vi "Log Messages.vi"(8 "error in (no error)":errorcluster, 10 "Actor to Log":refnum<class "Message Enqueuer.lvclass">, 11 "Monitor in":refnum<class "Classic Monitor.lvclass">) -> (0 "error out":errorcluster, 3 "Monitor out":refnum<class "Classic Monitor.lvclass">)   [LabVIEW 2023, in "Monitored Actor.lvlib" / "Classic Monitor.lvclass"]
doc: "Starts message logging on the specified actor\n\nCopyright: MGI 2016\nAuthor: Derek Trepanier"
uses:
  Classic Monitor.lvclass
  C:/Users/Public/Documents/Development/Framework/Monitored Actor/Actor Monitor/Actor Monitor/Actor Monitor.lvclass
  C:/Users/Public/Documents/Development/builds/Framework/Actor Framework.lvlibp/1abvi3w/vi.lib/ActorFramework/Actor/Actor.lvclass
  builds/Framework/Actor Framework.lvlibp/1abvi3w/vi.lib/ActorFramework/Message Enqueuer/Message Enqueuer.lvclass
  Actor Monitor/Actor Monitor/Actor Monitor.lvclass/Actor Monitor.ctl
  Classic Monitor.lvclass/Classic Monitor.ctl
  Logger/Classic Logger Actor/Classic Logger.lvclass
  Monitor Data/Monitor Data.lvclass
  Actor Monitor/Actor Monitor/Actor Monitor.lvclass
  Logger/Classic Logger Messages/Start Logging Msg/Start Logging Msg.lvclass
  builds/Framework/Actor Framework.lvlibp/1abvi3w/vi.lib/ActorFramework/Actor/Actor.lvclass
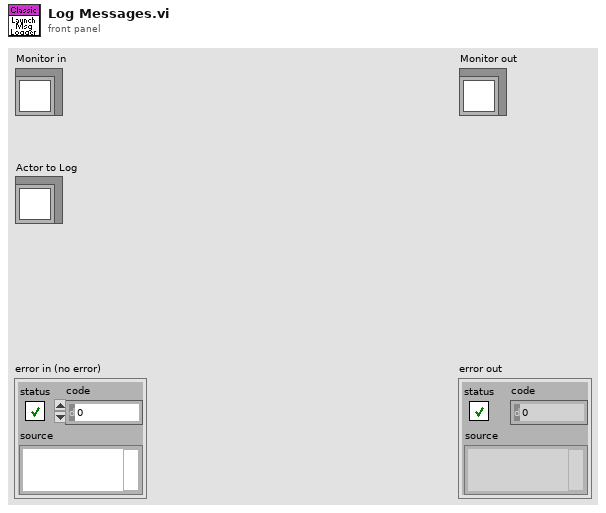
[diagram p1: front panel]
types:
  T1 = typedef "Monitored Actor.lvlib/Monitor Data.lvclass/Actor Data.ctl" = cluster{"Actor Type":string, "Actor Core VI":string, "Self":refnum<class "Message Enqueuer.lvclass">, "Caller":refnum<class "Message Enqueuer.lvclass">, "Actor Label":string, "Last Ping":dbl}
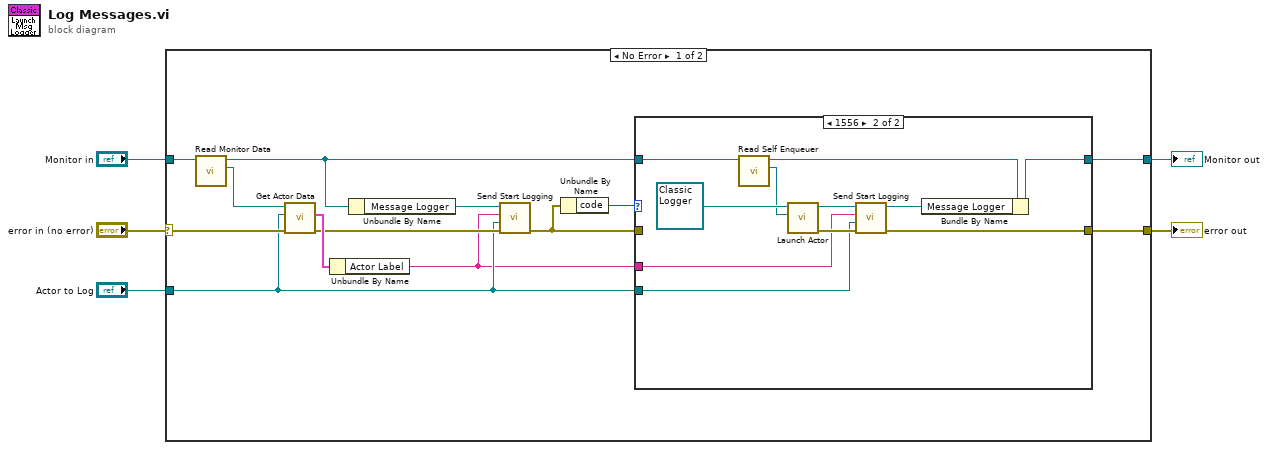
[diagram p0: block diagram]
diagram:
  n1 = case shown="No Error" "error in (no error)" {
    selector: "error in (no error)" -> [w15 w32]
    tunnel: [w16 w32] -> w4
    tunnel: [w18 w31] -> w2
    tunnel: "Monitor in" -> [w17 w31]
    tunnel: "Actor to Log" -> [w8 _]
    frame No Error {
      n2 = call "Read Monitor Data.vi"("Actor Monitor New in"=w17) -> ("Monitored Actor.lvlib:Monitor Data.lvclass"=w14:refnum<class "Monitor Data.lvclass">, "Actor Monitor New out"=w6:refnum<class "Classic Monitor.lvclass">)  [unwired: 8 in, 1 out]
      n3 = call "Get Actor Data.vi"("error in (no error)"=w15, "Actor's Self Q"=w8, "Monitor Data in"=w14) -> ("error out"=w10:errorcluster, "Actor Data"=w13:T1)  [unwired: 4 in, 3 out]
      n4 = Unbundle By Name(w13) -> ("Actor Label"=w7:string)
      n5 = Unbundle By Name(w6) -> ("Message Logger"=w11:refnum<class "Message Enqueuer.lvclass">)
      n6 = call "Send Start Logging.vi"("error in (no error)"=w10, "Actor to Log"=w8, "Label"=w7, "Message Enqueuer in"=w11) -> ("error out"=w9:errorcluster)  [unwired: 6 in, 1 out]
      n7 = Unbundle By Name(w9) -> ("code"=w12:i32)
      n8 = case shown="1556" w12 {
        tunnel: [w20 w30] -> w18
        tunnel: w6 -> [w20 w28]
        tunnel: w8 -> [_ w22]
        tunnel: w7 -> [_ w21]
        tunnel: [w19 w23] -> w16
        tunnel: w9 -> [w19 _]
        frame Default {
        }
        frame 1556 {
          n9 = call "Read Self Enqueuer.vi"("Actor"=w28) -> ("Self Enqueuer"=w27:refnum<class "Message Enqueuer.lvclass">)  [unwired: 10 in]
          n10 = call "Launch Actor.vi"("Actor-to-Caller Enqueuer"=w27, "Actor"=refnum<class "Classic Logger.lvclass"> refnum ("Classic Monitor.lvlib:Message Logger.lvclass")) -> ("error out"=w26:errorcluster, "Caller-To-Actor Enqueuer"=w25:refnum<class "Message Enqueuer.lvclass">)  [unwired: 8 in]
          n11 = call "Send Start Logging.vi"("error in (no error)"=w26, "Actor to Log"=w22, "Label"=w21, "Message Enqueuer in"=w25) -> ("error out"=w23:errorcluster, "Message Enqueuer out"=w24:refnum<class "Message Enqueuer.lvclass">)  [unwired: 6 in]
          n12 = Bundle By Name(cluster=w28, "Message Logger"=w24) -> (w30:refnum<class "Classic Monitor.lvclass">)
        }
      }
    }
    frame Error {
    }
  }
  "error out" <- w4
  "Monitor out" <- w2
